vi "BoolStatus.vi"(8 "错误输入（无错误）":errorcluster, 10 "Resultdata":T1={"Pressure"=0.0, "Pressure Boole"=TRUE, "Flow"=0.0, "Flow Boole"=TRUE, "Status"="Waiting"} {"Flow" format="%#_13g"; "Pressure" format="%#_13g"}, 11 "Result":refnum<vi>) -> (0 "error out":errorcluster caption="错误输出")   [LabVIEW 2017]
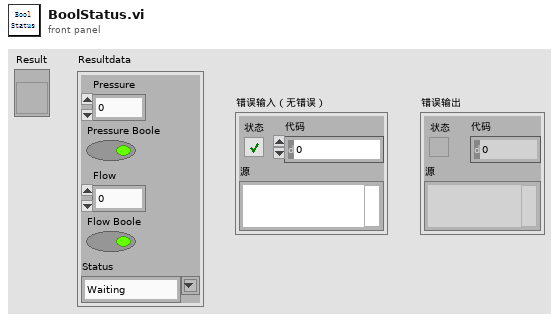
[diagram p1: front panel]
types:
  T1 = cluster{"Pressure":dbl, "Pressure Boole":bool, "Flow":dbl, "Flow Boole":bool, "Status":string}
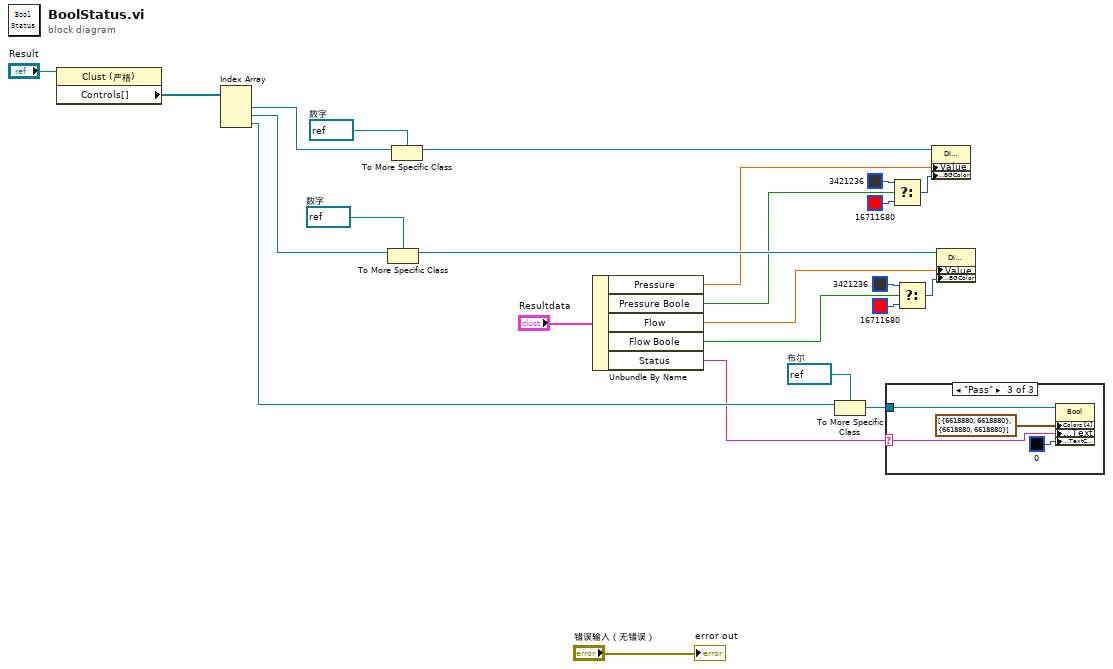
[diagram p0: block diagram]
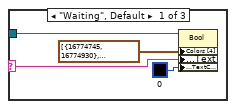
[diagram p2: hidden frame]
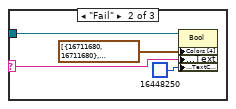
[diagram p3: hidden frame]
diagram:
  w10 = refnum<vi> refnum  # 数字
  w20 = refnum<vi> refnum  # 数字
  w23 = refnum<vi> refnum  # 布尔
  n1 = property class="Clust (严格)"(reference="Result") -> ("Controls[]"=w24:refnum<vi>[])  [unwired: 1 in, 2 out]
  n2 = Index Array(array=w24) -> (element #1=w18:refnum<vi>, element #2=w9:refnum<vi>, element #3=w21:refnum<vi>)  [unwired: 3 in]
  n3 = To More Specific Class(target class=w10, reference=w9) -> (specific class reference=w11:refnum<vi>)  [unwired: 1 in, 1 out]
  n4 = To More Specific Class(target class=w20, reference=w18) -> (specific class reference=w19:refnum<vi>)  [unwired: 1 in, 1 out]
  n5 = Unbundle By Name("Resultdata") -> ("Pressure"=w6:dbl, "Pressure Boole"=w5:bool, "Flow"=w4:dbl, "Flow Boole"=w3:bool, "Status"=w2:string)
  n6 = To More Specific Class(target class=w23, reference=w21) -> (specific class reference=w22:refnum<vi>)  [unwired: 1 in, 1 out]
  n7 = case shown="\"Pass\"" w2 {
    selector: w2 -> [w25 w29 w33]
    tunnel: w22 -> [w27 w32 w35]
    frame "Waiting", Default {
      n8 = property on="属性节点" class="Bool"(reference=w27, "Colors [4]"=cluster{u32, u32}[] [{16774745, 16774930}, {16774745, 16776002}], "BoolText.Text"=w25, "BoolText.TextColor"=u32 0) -> ()  [unwired: 1 in, 2 out]
    }
    frame "Fail" {
      n9 = property on="属性节点" class="Bool"(reference=w32, "Colors [4]"=cluster{u32, u32}[] [{16711680, 16711680}, {16711680, 16711680}], "BoolText.Text"=w29, "BoolText.TextColor"=u32 16448250) -> ()  [unwired: 1 in, 2 out]
    }
    frame "Pass" {
      n10 = property on="属性节点" class="Bool"(reference=w35, "Colors [4]"=cluster{u32, u32}[] [{6618880, 6618880}, {6618880, 6618880}], "BoolText.Text"=w33, "BoolText.TextColor"=u32 0) -> ()  [unwired: 1 in, 2 out]
    }
  }
  n11 = Select(t=u32 3421236, s=w5, f=u32 16711680) -> (s? t:f=w15:u32)
  n12 = Select(t=u32 3421236, s=w3, f=u32 16711680) -> (s? t:f=w14:u32)
  n13 = property class="DigNum"(reference=w19, "Value"=w6, "NumText.BGColor"=w15) -> ()  [unwired: 1 in, 2 out]
  n14 = property class="DigNum"(reference=w11, "Value"=w4, "NumText.BGColor"=w14) -> ()  [unwired: 1 in, 2 out]
  "error out" <- "错误输入（无错误）"
